vi "Attitude Indicator Interface.vi"(11 "RPY-Array":cdb[][](array[numeric])) -> (1 "Attitude in radians":cluster{"Roll":dbl, "Pitch":dbl, "Yaw":dbl}, 3 "Attitude in degrees":cluster{"Roll":dbl, "Pitch":dbl, "Yaw":dbl})   [LabVIEW 2013]
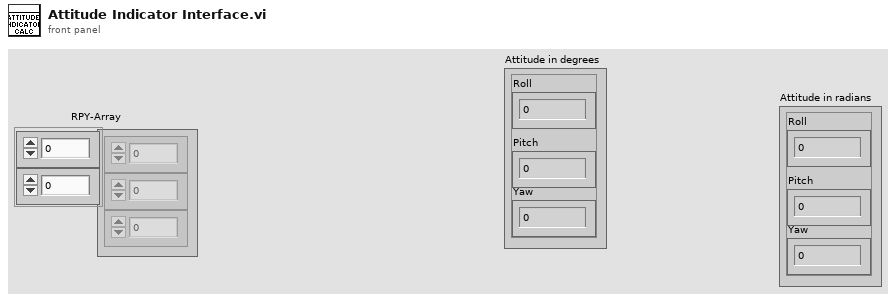
[diagram p1: front panel]
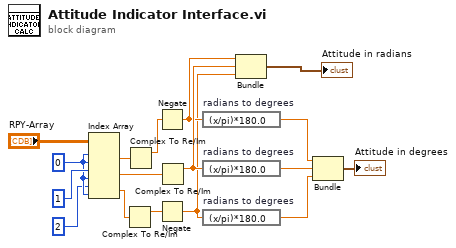
[diagram p0: block diagram]
diagram:
  w13 = 0 ("index (row)")
  n1 = Index Array(array="RPY-Array", index (row) #1=w13, index (col) #1=w13, index (row) #2=1 ("index (row)"), index (col) #2=w13, index (row) #3=2 ("index (row)"), index (col) #3=w13) -> (element #1=w16:cdb, element #2=w17:cdb, element #3=w11:cdb)
  n2 = Complex To Re/Im(x + iy=w11) -> (x=w7:dbl)  [unwired: 1 out]
  n3 = Complex To Re/Im(x + iy=w16) -> (x=w9:dbl)  [unwired: 1 out]
  n4 = Negate(x=w9) -> (-x=w2:dbl)
  n5 = Negate(x=w7) -> (-x=w1:dbl)
  n6 = Complex To Re/Im(x + iy=w17) -> (x=w8:dbl)  [unwired: 1 out]
  n7 = expression code="(x/pi)*180.0" "radians to degrees"(w2) -> (w3:dbl)
  n8 = expression code="(x/pi)*180.0" "radians to degrees"(w8) -> (w10:dbl)
  n9 = expression code="(x/pi)*180.0" "radians to degrees"(w1) -> (w6:dbl)
  n10 = Bundle(w2, w8, w1) -> (→"Attitude in radians":cluster{dbl, dbl, dbl})  [unwired: 1 in]
  n11 = Bundle(w3, w10, w6) -> (→"Attitude in degrees":cluster{dbl, dbl, dbl})  [unwired: 1 in]
